vi "Read CMD.vi"(8 "error in (no error)":errorcluster, 11 "Instr Actor in":refnum<class "Instr Actor.lvclass">) -> (0 "error out":errorcluster, 2 "CMD":refnum<queue>, 3 "Instr Actor out":refnum<class "Instr Actor.lvclass">)   [LabVIEW 2014, in "Instrument Library.lvlib" / "Instr Actor.lvclass"]
uses:
  Instr Actor.lvclass
  reusable/Command/Command.lvclass
  Instr Actor.lvclass/Instr Actor.ctl
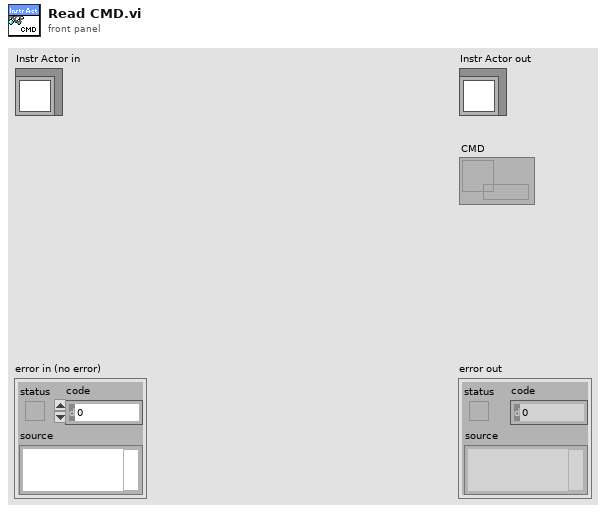
[diagram p1: front panel]
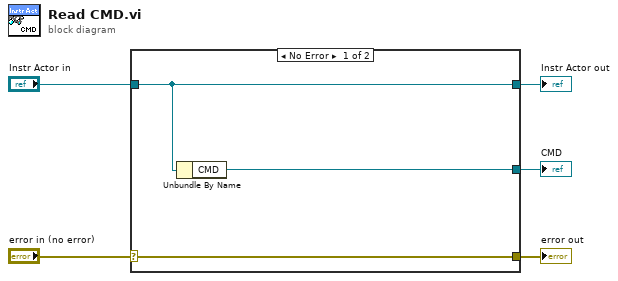
[diagram p0: block diagram]
diagram:
  n1 = case shown="No Error" "error in (no error)" {
    selector: "error in (no error)" -> [w8 w9]
    tunnel: [w8 w9] -> w4
    tunnel: [w7 w10] -> w2
    tunnel: "Instr Actor in" -> [w7 w10]
    tunnel: [w6 _] -> w1
    frame No Error {
      n2 = Unbundle By Name(w7) -> ("CMD"=w6:refnum<queue>)
    }
    frame Error {
    }
  }
  "error out" <- w4
  "Instr Actor out" <- w2
  "CMD" <- w1
